vi "FTW-ScripterStep-Wait-Core_Initialize.vi"(0 "Initialization Sequence":string, 5 "FTW Actor Instance Configuration":string, 11 "error in (no error)":errorcluster) -> (4 "FTW-ScripterStep-Wait-Core Out":refnum<class "FTW-ScripterStep-Wait-Core.lvclass">, 6 "Event Refnums":T1, 10 "Wait Time":dbl, 15 "error out":errorcluster)   [LabVIEW 2015, in "FTW-ScripterStep-Wait-Core.lvclass"]
uses:
  FTW-ScripterStep-Wait-Core.lvclass
  source/actor/Message/Request/FTW-Message-IncomingRequest.lvclass
  source/actor/Message/Base/FTW-Message.lvclass
  source/JSON/core/FTW-JSON-Core-EncodingFlags.vi
  source/JSON/FTW-JSON-Parse.vi
  source/Reflection/FTW-Reflection-Type.vi
  source/CodeGen/JSON Deserialize/FTW-JSON-Core-GetFlattenedValue.vi
  source/CodeGen/JSON Deserialize/FTW-JSON-Deserialize.xnode
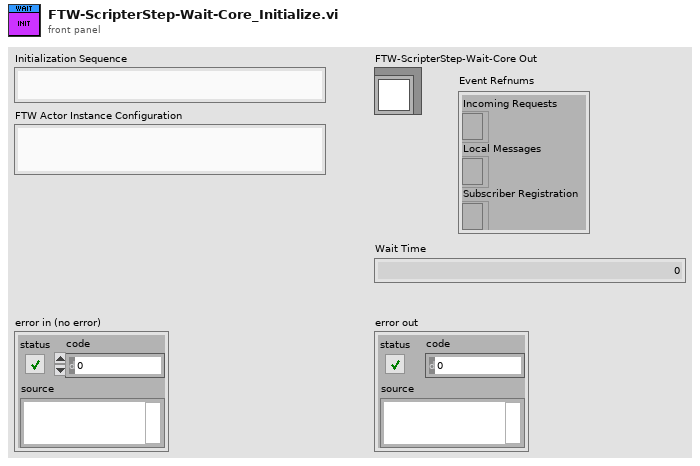
[diagram p1: front panel]
types:
  T1 = cluster{"Incoming Requests":refnum<event-registration>, "Local Messages":refnum<event-registration>, "Subscriber Registration":refnum<event-registration>}
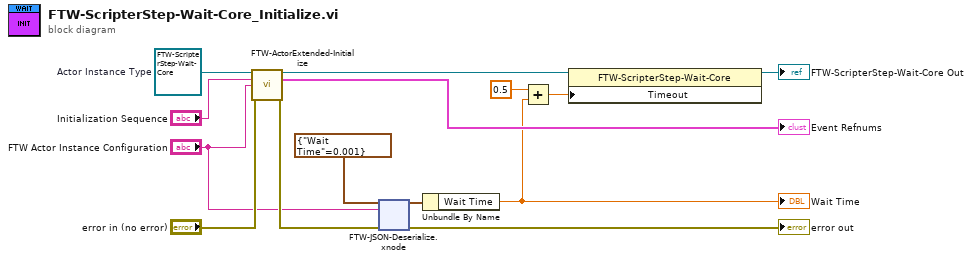
[diagram p0: block diagram]
diagram:
  w14 = refnum<class "FTW-ScripterStep-Wait-Core.lvclass"> refnum  # Actor Instance Type
  n1 = call-dynamic "FTW-ActorExtended-Initialize.vi"("FTW Actor Instance Type"=w14, "Initialization Job Sequence"="Initialization Sequence", "Actor Instance Configuration"="FTW Actor Instance Configuration", "error in"="error in (no error)") -> ("FTW Actor Instance"=w10:refnum<class "FTW-ScripterStep-Wait-Core.lvclass">, "Event Refnums"=→"Event Refnums":T1, "error out"=w8:errorcluster)  [unwired: 9 in]
  n2 = xnode "FTW-JSON-Deserialize.xnode"("Type and Defaults"=cluster{"Wait Time":dbl} {"Wait Time"=0.001}, "JSON String"="FTW Actor Instance Configuration", "error in"=w8) -> ("Values"=w11:cluster{"Wait Time":dbl}, "error out"=→"error out":errorcluster)
  n3 = Unbundle By Name(w11) -> ("Wait Time"=w3:dbl)
  "Wait Time" <- w3
  n4 = Add(x=0.5, y=w3) -> (x+y=w1:dbl)
  n5 = property class="FTW-ScripterStep-Wait-Core"(reference=w10, "Timeout"=w1) -> (reference out=→"FTW-ScripterStep-Wait-Core Out":refnum<class "FTW-ScripterStep-Wait-Core.lvclass">)  [unwired: 1 in, 1 out]
